vi "Write Single File Properties.vi"(8 "error in (no error)":errorcluster, 10 "File Properties in":T1, 11 "VI":refnum<vi>) -> (0 "error out":errorcluster, 3 "VI out":refnum<vi>)   [LabVIEW 2020, in "DocTool.lvlib"]
uses:
  DocTool.lvlib
  TDefs/Single File Properties.ctl
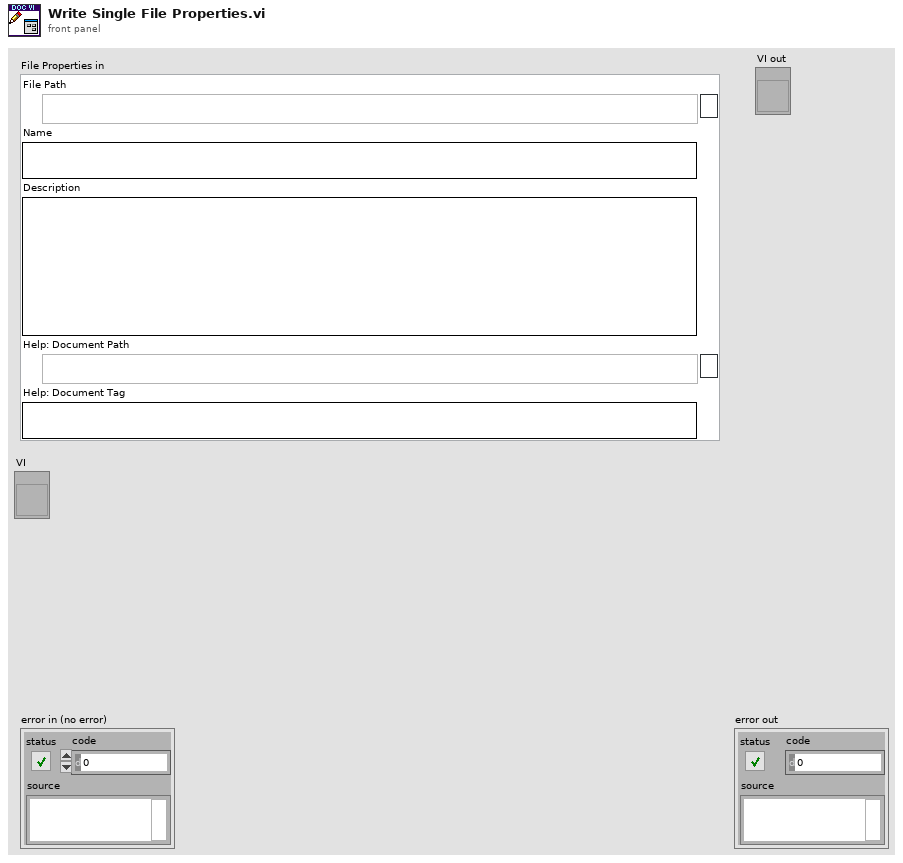
[diagram p1: front panel]
types:
  T1 = typedef "DocTool.lvlib/Single File Properties.ctl" = cluster{"File Path":path, "Name":string, "Description":string, "Help: Document Path":path, "Help: Document Tag":string}
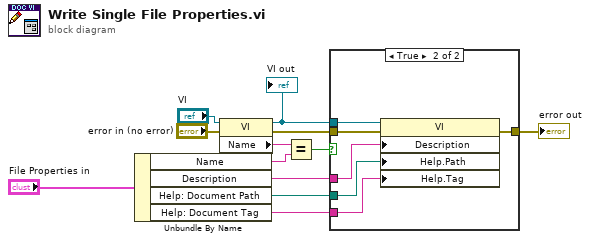
[diagram p0: block diagram]
diagram:
  n1 = Unbundle By Name("File Properties in") -> ("Name"=w3:string, "Description"=w8:string, "Help: Document Path"=w9:path, "Help: Document Tag"=w11:string)
  n2 = property class="VI"(reference="VI", error in="error in (no error)") -> (reference out=w5:refnum<vi>, error out=w6:errorcluster, "Name"=w2:string)
  "VI out" <- w5
  n3 = Equal?(x=w2, y=w3) -> (x = y?=w1:bool)
  n4 = case shown="True" w1 {
    tunnel: w11 -> [_ w19]
    tunnel: [w13 w18] -> w10
    tunnel: w9 -> [_ w17]
    tunnel: w8 -> [_ w16]
    tunnel: w6 -> [w13 w15]
    tunnel: w5 -> [_ w14]
    frame False {
    }
    frame True {
      n5 = property class="VI"(reference=w14, error in=w15, "Description"=w16, "Help.Path"=w17, "Help.Tag"=w19) -> (error out=w18:errorcluster)  [unwired: 1 out]
    }
  }
  "error out" <- w10
